vi "Open VI for Selected Item.vi"(8 "error in (no error)":errorcluster, 11 "Debugger In":refnum<class "Debugger.lvclass">) -> (0 "error out":errorcluster, 3 "Debugger Out":refnum<class "Debugger.lvclass">)   [LabVIEW 2020, in "Debugger.lvclass"]
uses:
  Debugger.lvclass
  C:/Users/anton/Documents/GitHub/triarc-debugger/source/Process/Debug Process.lvclass
  Process/Debug Process.lvclass/Debug Process.ctl
  Debugger.lvclass/Debugger.ctl
  Debug Log/Debug Log.lvclass/Debug Log.ctl
  Debug Data/Debug Data.lvclass/Debug Data.ctl
  <vilib>/Utility/error.llb/Clear Errors.vi
  <vilib>/Utility/error.llb/Error Cluster From Error Code.vi
  Process/Debug Process.lvclass
  Debug Log/Debug Log.lvclass
  Debug Data/Debug Data.lvclass
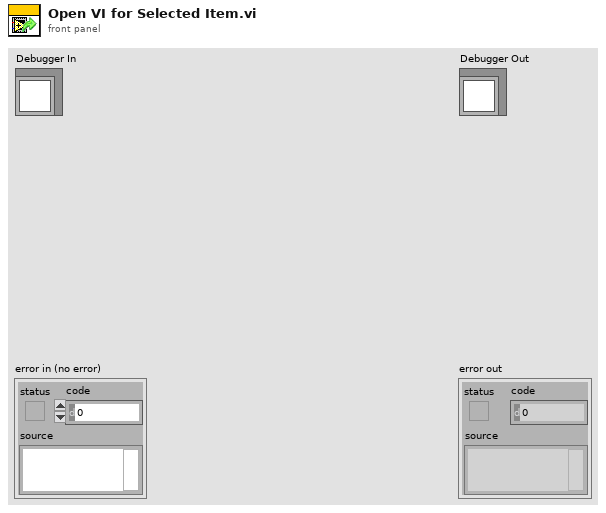
[diagram p1: front panel]
types:
  T1 = enum32{"Invalid", "Standard", "Closed", "Hidden", "Minimized", "Maximized"}
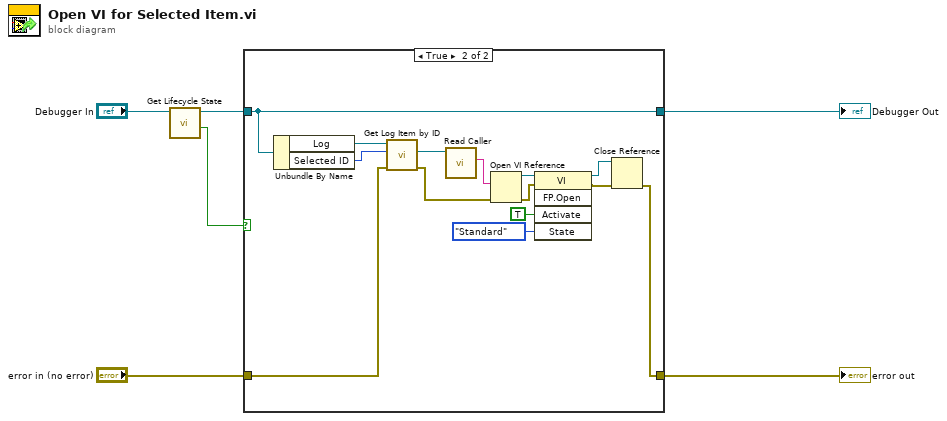
[diagram p0: block diagram]
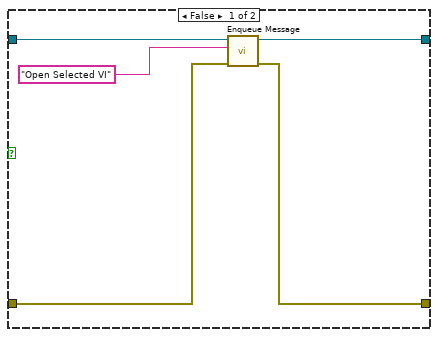
[diagram p2: hidden frame]
diagram:
  n1 = call "Get Lifecycle State.vi"("Process In"="Debugger In") -> ("In Process Loop?"=w1:bool, "Process Out"=w2:refnum<class "Debugger.lvclass">)  [unwired: 7 in, 2 out]
  n2 = case shown="True" w1 {
    tunnel: "error in (no error)" -> [w11 w23]
    tunnel: [w10 w15] -> w5
    tunnel: [w9 w22] -> w3
    tunnel: w2 -> [w7 w22]
    frame False {
      n3 = call "Enqueue Message.vi"("error in (no error)"=w11, "Message"="Open Selected VI", "Process In"=w7) -> ("error out"=w10:errorcluster, "Process Out"=w9:refnum<class "Debugger.lvclass">)  [unwired: 7 in]
    }
    frame True {
      n4 = Unbundle By Name(w22) -> ("Log"=w25:refnum<class "Debug Log.lvclass">, "Selected ID"=w24:u32)
      n5 = call "Get Log Item by ID.vi"("error in (no error)"=w23, "ID"=w24, "Debug Log In"=w25) -> ("error out"=w12:errorcluster, "Data Log"=w21:refnum<class "Debug Data.lvclass">)  [unwired: 6 in, 1 out]
      n6 = call "Read Caller.vi"("Debug Data in"=w21) -> ("Caller"=w16:string)  [unwired: 9 in, 1 out]
      n7 = Open VI Reference(vi path=w16, error in (no error)=w12) -> (vi reference=w19:refnum<vi>, error out=w17:errorcluster)  [unwired: 4 in]
      n8 = invoke class="VI" method="FP.Open"(reference=w19, error in=w17, "Activate"=TRUE ("Activate?"), "State"=T1."Standard") -> (reference out=w20:refnum<vi>, error out=w18:errorcluster)  [unwired: 1 in, 3 out]
      n9 = Close Reference(reference=w20, error in (no error)=w18) -> (error out=w15:errorcluster)
    }
  }
  "error out" <- w5
  "Debugger Out" <- w3
